vi "SetMatlabBoundControl.vi"(10 "Control Binding":T1, 11 "ExperimentID":string) -> ()   [LabVIEW 2017]
uses:
  Types/ControlValueChangeEventBindingType.ctl
  Types/MatlabBindingDirectionEnum.ctl
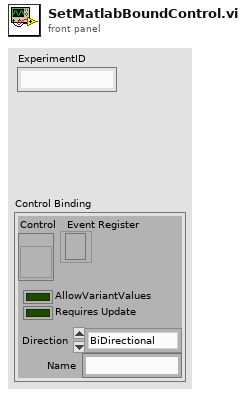
[diagram p1: front panel]
types:
  T1 = typedef "ControlValueChangeEventBindingType.ctl" = cluster{"Control":refnum<vi>, "Event Register":refnum<event-registration>, "AllowVariantValues":bool, "Direction":T2, "Requires Update":bool, "Name":string}
  T2 = typedef "MatlabBindingDirectionEnum.ctl" = enum16{"BiDirectional", "FromMatlab", "ToMatlab"}
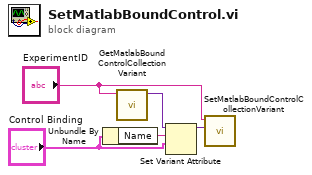
[diagram p0: block diagram]
diagram:
  n1 = Unbundle By Name("Control Binding") -> ("Name"=w1:string)
  n2 = call "GetMatlabBoundControlCollectionVariant.vi"("ExpID"="ExperimentID") -> ("BoundControlCollectionVariant"=w5:variant)  [unwired: 10 in]
  n3 = Set Variant Attribute(Variant=w5, name=w1, value="Control Binding") -> (Variant out=w4:variant)  [unwired: 1 in, 2 out]
  n4 = call "SetMatlabBoundControlCollectionVariant.vi"("BoundControlCollectionVariant in"=w4, "ExpID"="ExperimentID") -> ()  [unwired: 9 in, 1 out]
